vi "Main.vi"() -> ()   [LabVIEW 2021]
uses:
  <vilib>/vision/driver/NI_Vision_Acquisition_Software.lvlib
panel:
  out "Image":T1(plugin-control)
  in  "Camera Name":refnum<k21> caption="IMAQdx Session"
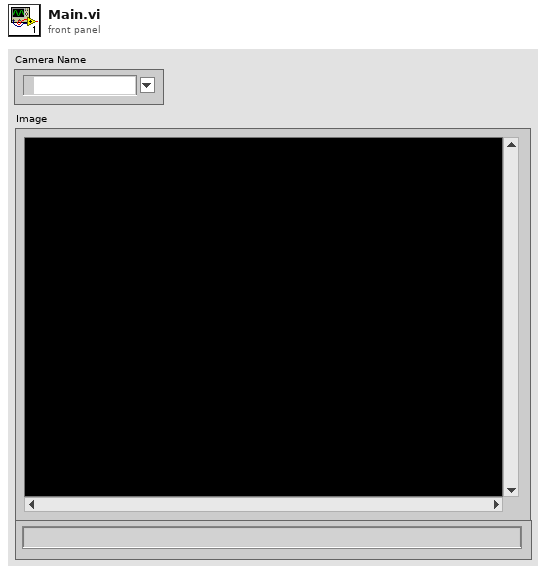
[diagram p1: front panel]
types:
  T1 = typedef "IMAQ Image.ctl" = refnum<image>
  T2 = typedef "Image Type" = u32
  T3 = typedef "IMAQdx.ctl" = refnum<k21>
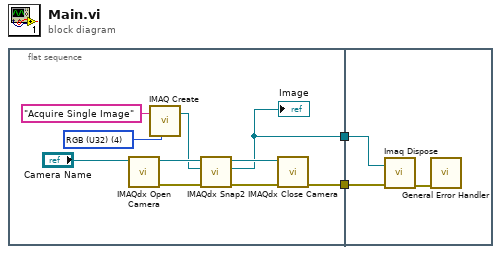
[diagram p0: block diagram]
diagram:
  n1 = flat-sequence {
    tunnel: [w11] -> w2
    tunnel: [w4] -> w1
    tunnel: w2 -> [w15]
    tunnel: w1 -> [w14]
    frame #0 {
      w3 = T2 4 items=["Grayscale (U8)", "Grayscale (I16)", "Grayscale (SGL)", "Complex (CSG)", "RGB (U32)", "HSL (U32)", "RGB (U64)", "Grayscale (U16)"] ("Image Type")
      n2 = call <vilib>:"IMAQdx Open Camera.vi"("Session In"="Camera Name") -> ("error out"=w7:errorcluster, "Session Out"=w10:T3)  [unwired: 2 in, 7 out]
      n3 = call "IMAQ Create"("Image Name"="Acquire Single Image", "Image Type"=w3) -> ("New Image"=w6:T1)  [unwired: 2 in, 2 out]
      n4 = call <vilib>:"IMAQdx Snap2.vi"("error in"=w7, "Image In"=w6, "Session In"=w10) -> ("error out"=w9:errorcluster, "Image Out"=w4:T1, "Session Out"=w12:T3)  [unwired: 6 in]
      "Image" <- w4
      n5 = call <vilib>:"IMAQdx Close Camera.vi"("error in"=w9, "Session In"=w12) -> ("error out"=w11:errorcluster)  [unwired: 9 out]
    }
    frame #1 {
      n6 = call "Imaq Dispose"("Image"=w14, "error in (no error)"=w15) -> ("error out"=w13:errorcluster)  [unwired: 4 in]
      n7 = call <vilib>:"General Error Handler.vi"("error in (no error)"=w13) -> ()  [unwired: 2 in, 13 out]
    }
  }
